vi "Test Position Write.vi"() -> ()   [LabVIEW 2020, in "Terminal.lvlib" / "TermBuffer.lvclass"]
uses:
  TermBuffer.lvclass
  TermBuffer.lvclass/TermBuffer.ctl
panel:
  out "Picture":picture
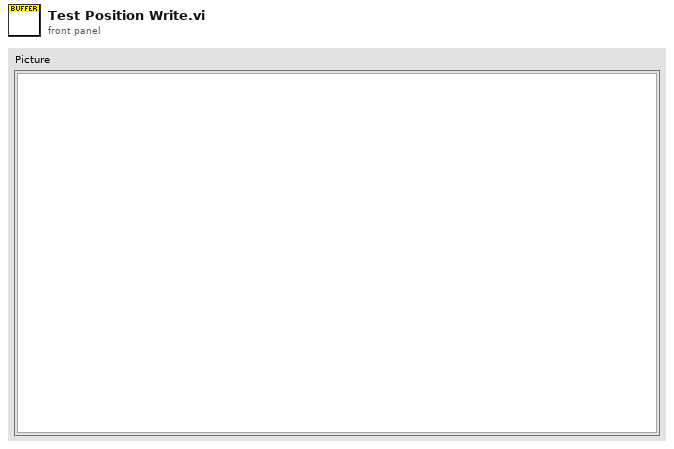
[diagram p1: front panel]
types:
  T1 = cluster{"Font Name:":string, "Size":i16, "Strikeout?":bool, "Italic?":bool, "Underline?":bool, "Outline?":bool, "Shadow?":bool, "Bold?":bool}
  T2 = enum16{"User-specified Font", "Application Font", "System Font", "Dialog Font"}
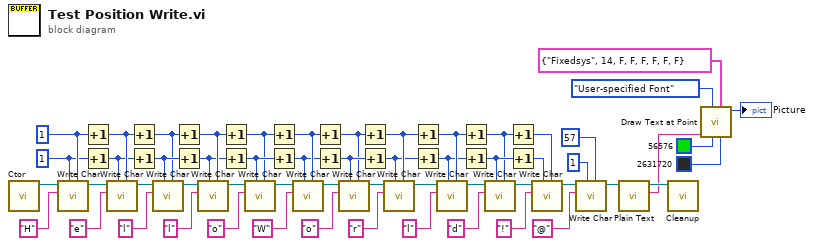
[diagram p0: block diagram]
diagram:
  w54 = 1 ("Col")
  w53 = 1 ("Row")
  n1 = call "Ctor.vi"() -> ("TermBuffer out"=w56:refnum<class "TermBuffer.lvclass">)  [unwired: 10 in, 1 out]
  n2 = call "Write Char.vi"("Col"=w54, "Row"=w53, "Char"="H", "TermBuffer in"=w56) -> ("TermBuffer out"=w52:refnum<class "TermBuffer.lvclass">)  [unwired: 6 in, 1 out]
  n3 = Increment(x=w54) -> (x+1=w39:i32)
  n4 = Increment(x=w53) -> (x+1=w38:i32)
  n5 = call "Write Char.vi"("Col"=w39, "Row"=w38, "Char"="e", "TermBuffer in"=w52) -> ("TermBuffer out"=w13:refnum<class "TermBuffer.lvclass">)  [unwired: 6 in, 1 out]
  n6 = Increment(x=w39) -> (x+1=w36:i32)
  n7 = Increment(x=w38) -> (x+1=w37:i32)
  n8 = call "Write Char.vi"("Col"=w36, "Row"=w37, "Char"="l", "TermBuffer in"=w13) -> ("TermBuffer out"=w14:refnum<class "TermBuffer.lvclass">)  [unwired: 6 in, 1 out]
  n9 = Increment(x=w36) -> (x+1=w35:i32)
  n10 = Increment(x=w37) -> (x+1=w34:i32)
  n11 = call "Write Char.vi"("Col"=w35, "Row"=w34, "Char"="l", "TermBuffer in"=w14) -> ("TermBuffer out"=w15:refnum<class "TermBuffer.lvclass">)  [unwired: 6 in, 1 out]
  n12 = Increment(x=w35) -> (x+1=w32:i32)
  n13 = Increment(x=w34) -> (x+1=w33:i32)
  n14 = call "Write Char.vi"("Col"=w32, "Row"=w33, "Char"="o", "TermBuffer in"=w15) -> ("TermBuffer out"=w16:refnum<class "TermBuffer.lvclass">)  [unwired: 6 in, 1 out]
  n15 = Increment(x=w32) -> (x+1=w31:i32)
  n16 = Increment(x=w33) -> (x+1=w30:i32)
  n17 = call "Write Char.vi"("Col"=w31, "Row"=w30, "Char"="W", "TermBuffer in"=w16) -> ("TermBuffer out"=w17:refnum<class "TermBuffer.lvclass">)  [unwired: 6 in, 1 out]
  n18 = Increment(x=w31) -> (x+1=w28:i32)
  n19 = Increment(x=w30) -> (x+1=w29:i32)
  n20 = call "Write Char.vi"("Col"=w28, "Row"=w29, "Char"="o", "TermBuffer in"=w17) -> ("TermBuffer out"=w18:refnum<class "TermBuffer.lvclass">)  [unwired: 6 in, 1 out]
  n21 = Increment(x=w28) -> (x+1=w27:i32)
  n22 = Increment(x=w29) -> (x+1=w26:i32)
  n23 = call "Write Char.vi"("Col"=w27, "Row"=w26, "Char"="r", "TermBuffer in"=w18) -> ("TermBuffer out"=w19:refnum<class "TermBuffer.lvclass">)  [unwired: 6 in, 1 out]
  n24 = Increment(x=w27) -> (x+1=w25:i32)
  n25 = Increment(x=w26) -> (x+1=w24:i32)
  n26 = call "Write Char.vi"("Col"=w25, "Row"=w24, "Char"="l", "TermBuffer in"=w19) -> ("TermBuffer out"=w20:refnum<class "TermBuffer.lvclass">)  [unwired: 6 in, 1 out]
  n27 = Increment(x=w25) -> (x+1=w22:i32)
  n28 = Increment(x=w24) -> (x+1=w23:i32)
  n29 = call "Write Char.vi"("Col"=w22, "Row"=w23, "Char"="d", "TermBuffer in"=w20) -> ("TermBuffer out"=w21:refnum<class "TermBuffer.lvclass">)  [unwired: 6 in, 1 out]
  n30 = Increment(x=w22) -> (x+1=w41:i32)
  n31 = Increment(x=w23) -> (x+1=w40:i32)
  n32 = call "Write Char.vi"("Col"=w41, "Row"=w40, "Char"="!", "TermBuffer in"=w21) -> ("TermBuffer out"=w5:refnum<class "TermBuffer.lvclass">)  [unwired: 6 in, 1 out]
  n33 = call "Write Char.vi"("Col"=57 ("Row"), "Row"=1, "Char"="@", "TermBuffer in"=w5) -> ("TermBuffer out"=w3:refnum<class "TermBuffer.lvclass">)  [unwired: 6 in, 1 out]
  n34 = call "Plain Text.vi"("TermBuffer in"=w3) -> ("Contents"=w8:string, "TermBuffer out"=w12:refnum<class "TermBuffer.lvclass">)  [unwired: 8 in, 1 out]
  n35 = call "Cleanup.vi"("TermBuffer in"=w12) -> ()  [unwired: 10 in, 1 out]
  n36 = call <vilib>:"Draw Text at Point.vi"("BG color(transparent)"=u32 2631720 ("text color(black)"), "[user-specified font]"=T1 {"Font Name:"="Fixedsys", "Size"=14, "Strikeout?"=FALSE, "Italic?"=FALSE, "Underline?"=FALSE, "Outline?"=FALSE, "Shadow?"=FALSE, "Bold?"=FALSE}, "text color(black)"=u32 56576, "desired font(Application)"=T2."User-specified Font", "text"=w8) -> ("new picture"=→"Picture":picture)  [unwired: 5 in, 1 out]
